vi "mxwScript_API_XMLRunVIOnObject.vi"(5 "modifyStack":bool, 6 "control values":T1[](array[typedef]), 7 "context":T2, 8 "error in (no error)":errorcluster, 9 "synchronous?":bool=TRUE, 10 "VI path":path, 11 "object name":string) -> (0 "error out":errorcluster, 3 "parameter":T1)   [LabVIEW 2017]
doc: "Create encoded control name for connecting to a terminal on a generic node instead of to a control terminal. Terminal is specified by name. If multiple terminals with the same name exist, the first one is used.\n\nThis encoding works for both connected to and connected from terminals."
uses:
  codeGenAPISupport.llb/cgAPI_mxwScript_Parameter.ctl
  codeGenAPISupport.llb/cgAPI_mxwScript_RunContext.ctl
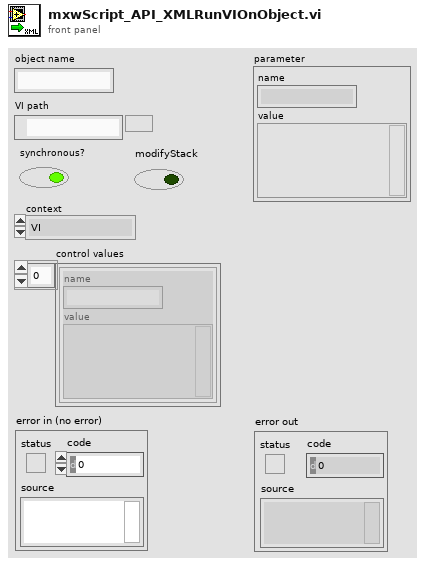
[diagram p1: front panel]
types:
  T1 = typedef "cgAPI_mxwScript_Parameter.ctl" = cluster{"name":string, "value":variant}
  T2 = typedef "cgAPI_mxwScript_RunContext.ctl" = enum16{"VI", "Engine"}
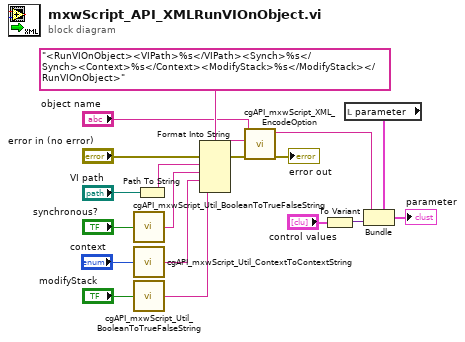
[diagram p0: block diagram]
diagram:
  n1 = call "cgAPI_mxwScript_Util_BooleanToTrueFalseString.vi"("boolean"="synchronous?") -> ("TRUE/FALSE text"=w1:string)  [unwired: 4 out]
  n2 = call "cgAPI_mxwScript_Util_ContextToContextString.vi"("context"="context") -> ("contextString"=w5:string)  [unwired: 4 out]
  n3 = call "cgAPI_mxwScript_Util_BooleanToTrueFalseString.vi"("boolean"="modifyStack") -> ("TRUE/FALSE text"=w3:string)  [unwired: 4 out]
  n4 = Path To String(path="VI path") -> (string=w8:string)
  n5 = Format Into String(format string="<RunVIOnObject><VIPath>%s</VIPath><Synch>%s</Synch><Context>%s</Context><ModifyStack>%s</ModifyStack></RunVIOnObject>" ("control name"), error in="error in (no error)", w8, w1, w5, w3) -> (resulting string=w15:string, error out=w17:errorcluster)  [unwired: 1 in]
  n6 = call "cgAPI_mxwScript_XML_EncodeOption.vi"("error in (no error)"=w17, "otherXML"=w15, "normalTextString"="object name") -> ("error out"=→"error out":errorcluster, "encodedString"=w9:string)  [unwired: 7 out]
  n7 = To Variant(anything="control values") -> (Variant=w11:variant)
  n8 = local read "parameter"() -> (w7:T1)
  n9 = Bundle(cluster=w7, "name"=w9, "value"=w11) -> (→"parameter":T1)
